vi "PH_IEEE1394Camera.destructor.vi"(0 "i ref in":refnum<vi>, 5 "error in(no error)":errorcluster) -> (19 "error out":errorcluster)   [LabVIEW 2014, in "PH_IEEE1394Camera.lvlib"]
doc: "This is the destructor of a class.\n\nLicense Agreement for this software:\n\nCopyright (C)\nGesellschaft für Schwerionenforschung, GSI\nPlanckstr. 1\n64291 Darmstadt\nGermany\n\nContact: D.Beck@gsi.de \n\nThis program is free software; you can redistribute it and/or modify it under the terms of the \nGNU General Public License as published by the Free Software Foundation; either version 2 of \nthe license, or (at your option) any later version.\n\nThis program is distributed in the hope that it will be useful, but WITHOUT ANY WARRANTY; \nwithout even the implied warranty of MERCHANTABILITY or FITNESS FOR A PARTICULAR PURPOSE. See the GNU General License for more details (http://www.gnu.org).\n\nGesellschaft für Schwerionenforschung, GSI\nPlanckstr. 1, 64291 Darmstadt, Germany\nFor all questions and ideas contact: M.Richter@gsi.de, H.Brand@gsi.de or D.Beck@gsi.de.\nLast update: 16-JUN-2004"
uses:
  PH_IEEE1394Camera.lvlib
  PH_Basics/PH_Cam_BaseClass/PH_Cam_BaseClass.lvlib
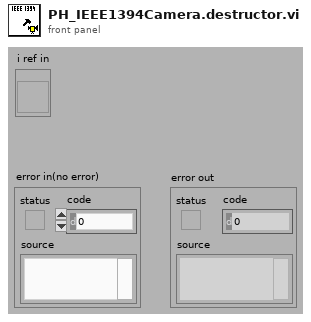
[diagram p1: front panel]
types:
  T1 = enum16{"SetAttribute", "GetAttribute", "CreateAttribute", "DestroyAttribute", "DestroyAllAtributes"}
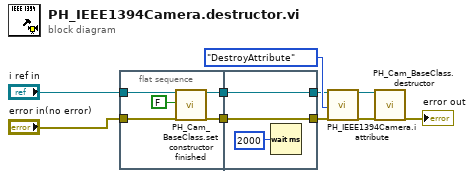
[diagram p0: block diagram]
diagram:
  n1 = flat-sequence {
    tunnel: "error in(no error)" -> [w12]
    tunnel: "i ref in" -> [w13]
    tunnel: [w11] -> w9
    tunnel: [w14] -> w8
    tunnel: [w17] -> w7
    tunnel: [w18] -> w6
    tunnel: w9 -> [w18]
    tunnel: w8 -> [w17]
    frame #0 {
      n2 = call "PH_Cam_BaseClass.set constructor finished.vi"("i ref in"=w13, "Contructor finished"=FALSE, "error in (no error)"=w12) -> ("i ref out"=w14:refnum<vi>, "error out"=w11:errorcluster)  [unwired: 15 in]
    }
    frame #1 {
      n3 = Wait (ms)(milliseconds to wait=u32 2000) -> ()  [unwired: 1 out]
    }
  }
  n4 = call "PH_IEEE1394Camera.i attribute.vi"("VI Refnum"=w7, "Action"=T1."DestroyAttribute", "error in (no error)"=w6) -> ("VI Refnum out"=w2:refnum<vi>, "error out"=w5:errorcluster)  [unwired: 14 in, 1 out]
  n5 = call "PH_Cam_BaseClass.destructor.vi"("i ref in"=w2, "error in(no error)"=w5) -> ("error out"=→"error out":errorcluster)  [unwired: 17 in]
